vi "czytajI2C.vi"(7 "I2C Channel":u8, 8 "Error In":errorcluster, 10 "I2C Slave Address (0x1D)":u8, 11 "LINX Resource in":T1) -> (0 "Error Out":errorcluster, 2 "Acceleration Data (g)":T7, 3 "LINX Resource out":T1)   [LabVIEW 2014]
uses:
  <vilib>/MakerHub/LINX/Private/Type Defs/LINX Ref.ctl
  <vilib>/MakerHub/LINX/Private/Type Defs/Platform.ctl
  <vilib>/MakerHub/LINX/Private/Type Defs/Interface.ctl
  <vilib>/MakerHub/LINX/Private/Device/Type Defs/LINX Device Config.ctl
  <vilib>/MakerHub/LINX/Private/Device/Type Defs/TCP Config.ctl
  <vilib>/MakerHub/LINX/Private/Device/Type Defs/Channels.ctl
  <vilib>/MakerHub/LINX/Private/Local IO/LinxI2cWrite.vi
  <vilib>/MakerHub/LINX/Public/Utilities/Check Channel.vi
  <vilib>/MakerHub/LINX/Private/Local IO/Handle Errors.vi
  <vilib>/MakerHub/LINX/Private/Utilties/Generate Error.vi
  <vilib>/MakerHub/LINX/LMH-LINX.lvlib
  <vilib>/MakerHub/LINX/Private/Device/Device.lvlib
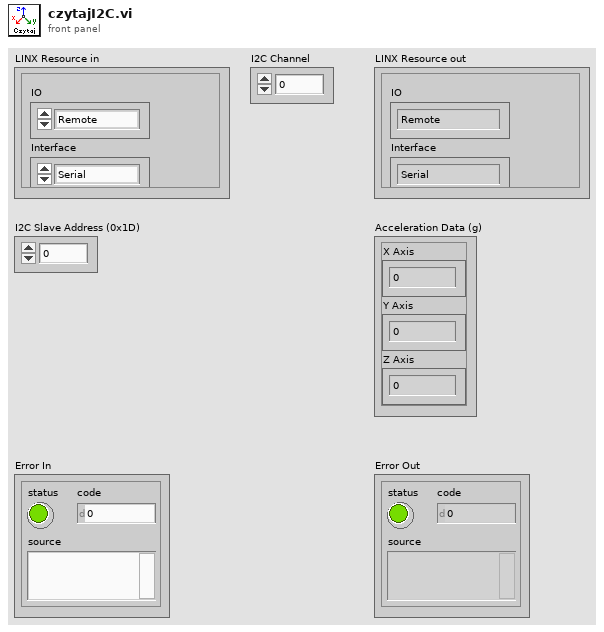
[diagram p1: front panel]
types:
  T1 = typedef "LMH-LINX.lvlib/LINX Ref.ctl" = cluster{"IO":T2, "Interface":T3, "LINX Device Config":T4}
  T2 = typedef "LMH-LINX.lvlib/Platform.ctl" = enum16{"Remote", "Local"}
  T3 = typedef "LMH-LINX.lvlib/Interface.ctl" = enum16{"Serial", "TCP"}
  T4 = typedef "LMH-LINX.lvlib/Device.lvlib/LINX Device Config.ctl" = cluster{"Interface":T3, "COM Port":refnum<visa-resource-name>, "TCP Configuration":T5, "Device Family":u8, "Device ID":u8, "Device Name":string, "TCP Ref":refnum<k5>, "Channels":T6}
  T5 = typedef "LMH-LINX.lvlib/Device.lvlib/TCP Config.ctl" = cluster{"IP Address":string, "Port":u16}
  T6 = typedef "LMH-LINX.lvlib/Channels.ctl" = cluster{"DI":u8[], "DO":u8[], "AI":u8[], "AO":u8[], "PWM":u8[], "QE":u8[], "UART":u8[], "I2C 2":u8[], "SPI":u8[], "CAN":u8[], "Servo":u8[], "AI Ref (V)":dbl, "AI Resolution (Bits)":u8, "AO Ref (V)":dbl, "AO Resolution (Bits)":u8}
  T7 = cluster{"X Axis":dbl, "Y Axis":dbl, "Z Axis":dbl}
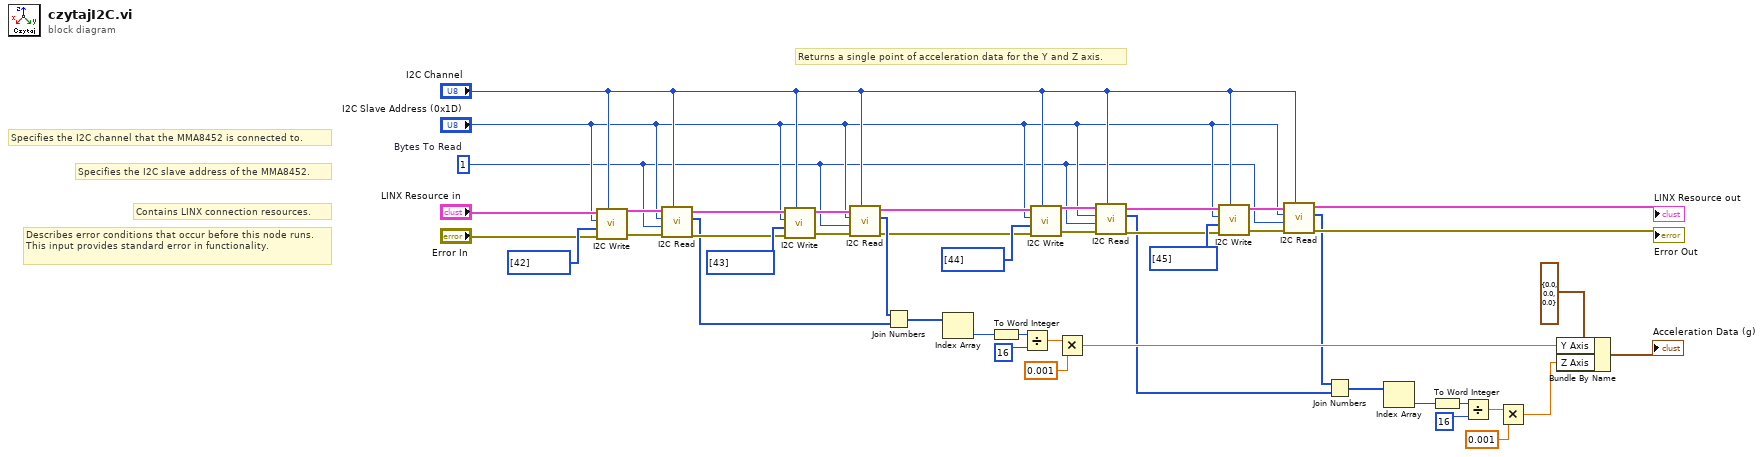
[diagram p0: block diagram]
diagram:
  w10 = u8 1  # Bytes To Read
  # "Returns a single point of acceleration data for the Y and Z axis."
  # "Specifies the I2C slave address of the MMA8452."
  # "Specifies the I2C channel that the MMA8452 is connected to."
  # "Contains LINX connection resources."
  # "Describes error conditions that occur before this node runs. This input provides standard error in functionality."
  n1 = call <vilib>:"I2C Write.vi"("I2C Channel"="I2C Channel", "Error In"="Error In", "Data"=u8[] [42], "I2C Slave Address (0)"="I2C Slave Address (0x1D)", "LINX Resource"="LINX Resource in") -> ("Error Out"=w43:errorcluster, "LINX Resource"=w44:T1)  [unwired: 5 in]
  n2 = call <vilib>:"I2C Read.vi"("I2C Channel"="I2C Channel", "Error In"=w43, "Bytes To Read"=w10, "I2C Slave Address (0)"="I2C Slave Address (0x1D)", "LINX Resource"=w44) -> ("Error Out"=w29:errorcluster, "Data"=w25:u8[], "LINX Resource"=w30:T1)  [unwired: 4 in]
  n3 = call <vilib>:"I2C Write.vi"("I2C Channel"="I2C Channel", "Error In"=w29, "Data"=u8[] [43], "I2C Slave Address (0)"="I2C Slave Address (0x1D)", "LINX Resource"=w30) -> ("Error Out"=w31:errorcluster, "LINX Resource"=w28:T1)  [unwired: 5 in]
  n4 = call <vilib>:"I2C Read.vi"("I2C Channel"="I2C Channel", "Error In"=w31, "Bytes To Read"=w10, "I2C Slave Address (0)"="I2C Slave Address (0x1D)", "LINX Resource"=w28) -> ("Error Out"=w15:errorcluster, "Data"=w26:u8[], "LINX Resource"=w16:T1)  [unwired: 4 in]
  n5 = Join Numbers(hi=w26, lo=w25) -> ((hi.lo)=w27:u16[])
  n6 = Index Array(array=w27) -> (element=w40:u16)  [unwired: 1 in]
  n7 = To Word Integer(number=w40) -> (16bit integer=w39:i16)
  n8 = Divide(x=w39, y=i16 16) -> (x/y=w37:dbl)
  n9 = call <vilib>:"I2C Write.vi"("I2C Channel"="I2C Channel", "Error In"=w15, "Data"=u8[] [44], "I2C Slave Address (0)"="I2C Slave Address (0x1D)", "LINX Resource"=w16) -> ("Error Out"=w22:errorcluster, "LINX Resource"=w23:T1)  [unwired: 5 in]
  n10 = Multiply(x=w37, y=0.001) -> (x*y=w35:dbl)
  n11 = call <vilib>:"I2C Read.vi"("I2C Channel"="I2C Channel", "Error In"=w22, "Bytes To Read"=w10, "I2C Slave Address (0)"="I2C Slave Address (0x1D)", "LINX Resource"=w23) -> ("Error Out"=w18:errorcluster, "Data"=w3:u8[], "LINX Resource"=w19:T1)  [unwired: 4 in]
  n12 = call <vilib>:"I2C Write.vi"("I2C Channel"="I2C Channel", "Error In"=w18, "Data"=u8[] [45], "I2C Slave Address (0)"="I2C Slave Address (0x1D)", "LINX Resource"=w19) -> ("Error Out"=w20:errorcluster, "LINX Resource"=w17:T1)  [unwired: 5 in]
  n13 = call <vilib>:"I2C Read.vi"("I2C Channel"="I2C Channel", "Error In"=w20, "Bytes To Read"=w10, "I2C Slave Address (0)"="I2C Slave Address (0x1D)", "LINX Resource"=w17) -> ("Error Out"=→"Error Out":errorcluster, "Data"=w2:u8[], "LINX Resource"=→"LINX Resource out":T1)  [unwired: 4 in]
  n14 = Join Numbers(hi=w2, lo=w3) -> ((hi.lo)=w4:u16[])
  n15 = Index Array(array=w4) -> (element=w9:u16)  [unwired: 1 in]
  n16 = To Word Integer(number=w9) -> (16bit integer=w8:i16)
  n17 = Divide(x=w8, y=i16 16) -> (x/y=w6:dbl)
  n18 = Multiply(x=w6, y=0.001) -> (x*y=w1:dbl)
  n19 = Bundle By Name(cluster=T7 {"X Axis"=0.0, "Y Axis"=0.0, "Z Axis"=0.0} ("Acceleration Data (g)"), "Y Axis"=w35, "Z Axis"=w1) -> (→"Acceleration Data (g)":T7)
